vi "Read PID Controller Values.vi"(7 "listen period":sgl=0.1, 8 "error in":errorcluster, 11 "Brooks MFC in":refnum<class "Brooks MFC.lvclass">) -> (0 "error out":errorcluster, 2 "PID":cluster{"Ki":sgl, "Kd":sgl, "Kp":sgl}={"Ki"=3.65, "Kd"=0.0, "Kp"=0.6}, 3 "Brooks MFC out":refnum<class "Brooks MFC.lvclass">)   [LabVIEW 2016, in "Brooks MFC.lvclass"]
uses:
  Brooks MFC.lvclass
  Brooks MFC.lvclass/Brooks MFC.ctl
  Instance           3 34Saved   Read PID Controller Values .vi
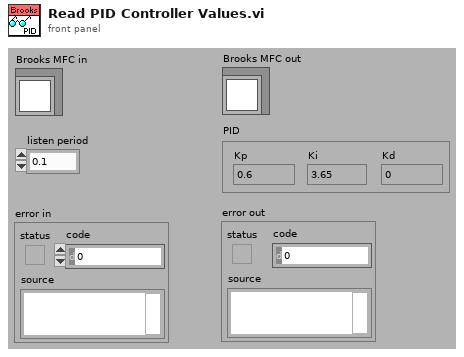
[diagram p1: front panel]
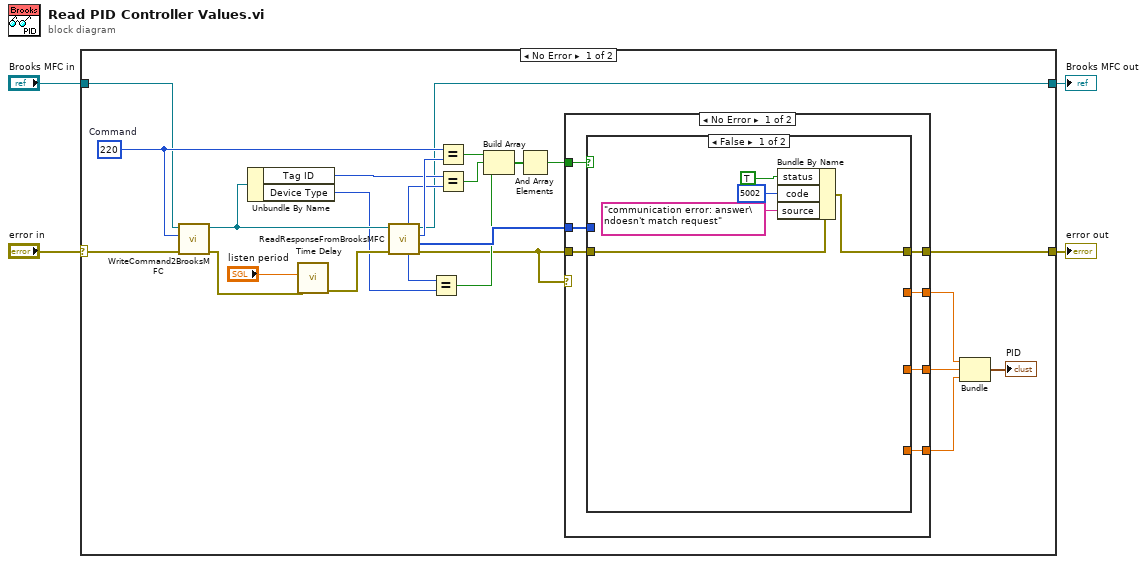
[diagram p0: block diagram]
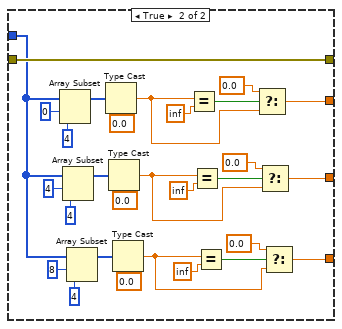
[diagram p2: hidden frame]
diagram:
  n1 = case shown="No Error" "error in" {
    selector: "error in" -> [w8 w72]
    tunnel: "Brooks MFC in" -> [w7 w73]
    tunnel: [w6 w73] -> w2
    tunnel: [w5 w72] -> w1
    frame No Error {
      w17 = u8 220  # Command
      n2 = call "WriteCommand2BrooksMFC.vi"("error in"=w8, "Command"=w17, "Brooks MFC in"=w7) -> ("error out"=w27:errorcluster, "Brooks MFC out"=w11:refnum<class "Brooks MFC.lvclass">)  [unwired: 6 in, 1 out]
      n3 = Unbundle By Name(w11) -> ("Tag ID"=w9:u32, "Device Type"=w10:u8)
      n4 = call "Time Delay"("error in (no error)"=w27, "Delay Time (s)"="listen period") -> ("error out"=w25:errorcluster)  [unwired: 9 in]
      n5 = call "ReadResponseFromBrooksMFC.vi"("error in"=w25, "Brooks MFC in"=w11) -> ("error out"=w12:errorcluster, "Data"=w29:u8[], "Command"=w28:u8, "Brooks MFC out"=w6:refnum<class "Brooks MFC.lvclass">, "device type"=w23:u8, "tag ID"=w24:u32)  [unwired: 4 in]
      n6 = Equal?(x=w23, y=w10) -> (x = y?=w20:bool)
      n7 = Equal?(x=w17, y=w28) -> (x = y?=w22:bool)
      n8 = Equal?(x=w9, y=w24) -> (x = y?=w21:bool)
      n9 = Build Array(w22, w21, w20) -> (w19:bool[])
      n10 = And Array Elements(Boolean array=w19) -> (logical AND=w18:bool)
      n11 = case shown="No Error" w12 {
        tunnel: w12 -> [w36 w71]
        tunnel: w29 -> [w35 _]
        tunnel: [w34 w71] -> w5
        tunnel: w18 -> [w33 _]
        tunnel: [w32 _] -> w15
        tunnel: [w31 _] -> w14
        tunnel: [w30 _] -> w13
        frame No Error {
          n12 = case shown="False" w33 {
            tunnel: w35 -> [_ w44]
            tunnel: w36 -> [w39 w68]
            tunnel: [w38 w68] -> w34
            tunnel: [_ w65] -> w32
            tunnel: [_ w52] -> w31
            tunnel: [_ w42] -> w30
            frame False {
              n13 = Bundle By Name(cluster=w39, "status"=TRUE ("Bundle Element"), "code"=5002 ("Bundle Element"), "source"="communication error: answer\ndoesn't match request") -> (w38:errorcluster)
            }
            frame True {
              n14 = Array Subset(array=w44, index=0 ("Array Index"), length=4 ("Array Length")) -> (w64:u8[])
              n15 = Array Subset(array=w44, index=4 ("Array Index"), length=4 ("Array Length")) -> (w56:u8[])
              n16 = Array Subset(array=w44, index=8 ("Array Index"), length=4 ("Array Length")) -> (w47:u8[])
              n17 = Type Cast(type=sgl 0.0 ("x"), x=w64) -> (*(type *) &x=w62:sgl)
              n18 = Type Cast(type=sgl 0.0 ("x"), x=w56) -> (*(type *) &x=w54:sgl)
              n19 = Type Cast(type=sgl 0.0 ("x"), x=w47) -> (*(type *) &x=w43:sgl)
              n20 = Equal?(x=w62, y=sgl inf ("Single")) -> (x = y?=w67:bool)
              n21 = Equal?(x=w54, y=sgl inf ("Single")) -> (x = y?=w58:bool)
              n22 = Equal?(x=w43, y=sgl inf ("Single")) -> (x = y?=w49:bool)
              n23 = Select(t=sgl 0.0 ("x"), s=w67, f=w62) -> (s? t:f=w65:sgl)
              n24 = Select(t=sgl 0.0 ("x"), s=w58, f=w54) -> (s? t:f=w52:sgl)
              n25 = Select(t=sgl 0.0 ("x"), s=w49, f=w43) -> (s? t:f=w42:sgl)
            }
          }
        }
        frame Error {
        }
      }
      n26 = Bundle("x"=w15, "x"=w14, "x"=w13) -> (→"PID":cluster{"x":sgl, "x":sgl, "x":sgl})  [unwired: 1 in]
    }
    frame Error {
    }
  }
  "Brooks MFC out" <- w2
  "error out" <- w1
